vi "Variant_FormatTreeItems.vi"(10 "Variant":variant) -> (2 "Tree Items":T1(array[cluster]))   [LabVIEW 2020, in "OpenVariant.lvlib"]
uses:
  OpenVariant.lvlib
  _built_ppls/OpenConvert.lvlibp
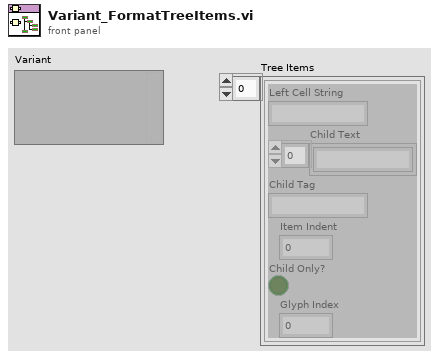
[diagram p1: front panel]
types:
  T1 = cluster{"Left Cell String":string, "Child Text":string[], "Child Tag":string, "Item Indent":i32, "Child Only?":bool, "Glyph Index":i32}[]
  T2 = cluster{"Left Cell String":string, "Child Text":string[], "Child Tag":string, "Item Indent":i32, "Child Only?":bool, "Glyph Index":i32}
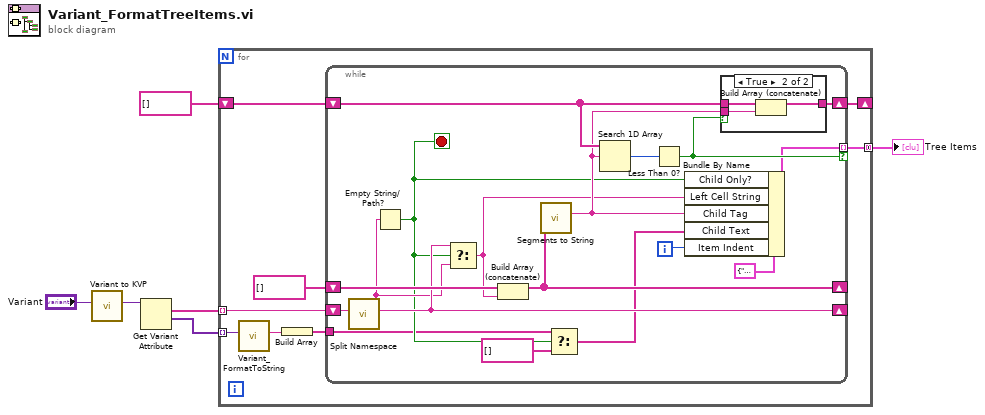
[diagram p0: block diagram]
diagram:
  n1 = call "Variant to KVP.vi"("Variant"="Variant") -> ("KVP Dictionary"=w6:variant)  [unwired: 10 in]
  n2 = Get Variant Attribute(Variant=w6) -> (names=w5:string[], values=w4:variant[])  [unwired: 3 in, 2 out]
  n3 = for {
    tunnel: w5 -> [w14] mode=indexing
    tunnel: w4 -> [w8] mode=indexing
    tunnel: [w12] -> w3 mode=concatenating
    shift-right: [w10] -> _
    shift-left: string[] [] -> [w11]
    n4 = call "Variant_FormatToString.vi"("Variant"=w8) -> ("Value"=w7:string)  [unwired: 10 in]
    n5 = Build Array(w7) -> (w9:string[])
    n6 = while {
      shift-right: [w30] -> _
      shift-left: string[] [] -> [w31]
      tunnel: [w17] -> w12 mode=indexing if=w18
      shift-right: [w26] -> _
      shift-left: w14 -> [w23]
      shift-right: [w27] -> w10
      shift-left: w11 -> [w28]
      tunnel: w9 -> [w21]
      i -> [w15]
      stop <- w22 stop-if-true
      n7 = call "Split Namespace.vi"("Namespaced String"=w23) -> ("String"=w26:string, "Namespace"=w24:string)  [unwired: 9 in]
      n8 = Empty String/Path?(string/path=w24) -> (empty?=w22:bool)
      n9 = Select(t=w26, s=w22, f=w24) -> (s? t:f=w16:string)
      n10 = Build Array (concatenate)(w31, w16) -> (w30:string[])
      n11 = call "Segments to String.vi"("Segments"=w30) -> ("String"=w25:string)  [unwired: 10 in]
      n12 = Select(t=w21, s=w22, f=string[] []) -> (s? t:f=w19:string[])
      n13 = Search 1D Array(1D array=w28, element=w25) -> (index of element=w29:i32)  [unwired: 1 in]
      n14 = Less Than 0?(x=w29) -> (x < 0?=w18:bool)
      n15 = Bundle By Name(cluster=T2 {"Left Cell String"="", "Child Text"=[], "Child Tag"="", "Item Indent"=0, "Child Only?"=FALSE, "Glyph Index"=0} ("Item"), "Child Only?"=w22, "Left Cell String"=w16, "Child Tag"=w25, "Child Text"=w19, "Item Indent"=w15) -> (w17:T2)
      n16 = case shown="True" w18 {
        tunnel: w28 -> [w33 w36]
        tunnel: w25 -> [_ w35]
        tunnel: [w33 w34] -> w27
        frame False {
        }
        frame True {
          n17 = Build Array (concatenate)(w36, w35) -> (w34:string[])
        }
      }
    }
  }
  "Tree Items" <- w3
